vi "niRFUtil FTW Generate RBW FIR Filter.vi"(0 "Type":T2=enum."Gaussian", 5 "Bandwidth (Hz)":T5=500000.0 format="%^.3e", 7 "Sampling Rate (Hz)":dbl=500000.0 format="%^.3e", 9 "Minimum Selectivity (dB)":dbl=70.0 format="%.2f", 11 "Alpha":T1=0.22 format="%.3g") -> (4 "Filter":T3 {"y" min=0 max=127 format="%.2f"; "dx" format="%^.2e"; "x0" format="%^.2e"})   [LabVIEW 2015, in "niRFUtil.lvlib"]
doc: "(c) Copyright 2006, National Instruments, Inc. This VI may not be duplicated, sold, or distributed without written consent from National Instruments."
uses:
  niRFUtil.lvlib
  Includes/niRFUtil INC RBW Filter Bandwidth.ctl
  Includes/niRFUtil INC Real Waveform.ctl
  Includes/niRFUtil INC Real Array.ctl
  Includes/niRFUtil INC RBW Filter Type (Time Domain).ctl
  Includes/niRFUtil INC RRC Filter Alpha.ctl
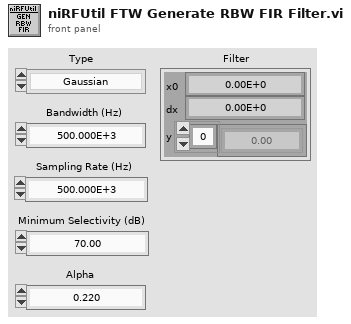
[diagram p1: front panel]
types:
  T1 = typedef "niRFUtil.lvlib/niRFUtil INC RRC Filter Alpha.ctl" = dbl
  T2 = typedef "niRFUtil.lvlib/niRFUtil INC RBW Filter Type (Time Domain).ctl" = enum16{"None", "Gaussian", "Flat", "Synch Tuned - 4", "Synch Tuned - 5", "RRC"}
  T3 = typedef "niRFUtil.lvlib/niRFUtil INC Real Waveform.ctl" = cluster{"x0":dbl, "dx":dbl, "y":T4}
  T4 = typedef "niRFUtil.lvlib/niRFUtil INC Real Array.ctl" = sgl[]
  T5 = typedef "niRFUtil.lvlib/niRFUtil INC RBW Filter Bandwidth.ctl" = dbl
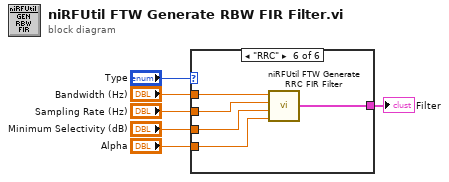
[diagram p0: block diagram]
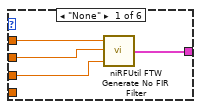
[diagram p2: hidden frame]
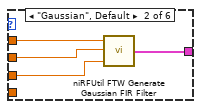
[diagram p3: hidden frame]
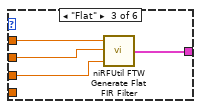
[diagram p4: hidden frame]
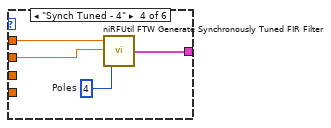
[diagram p5: hidden frame]
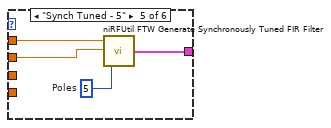
[diagram p6: hidden frame]
diagram:
  n1 = case shown="\"RRC\"" "Type" {
    tunnel: "Bandwidth (Hz)" -> [w10 w14 w18 w22 w26 w31]
    tunnel: "Sampling Rate (Hz)" -> [w9 w13 w17 w21 w25 w30]
    tunnel: "Minimum Selectivity (dB)" -> [w7 w12 w15 _ _ w29]
    tunnel: [w8 w11 w16 w20 w24 w27] -> w2
    tunnel: "Alpha" -> [_ _ _ _ _ w28]
    frame "None" {
      n2 = call "niRFUtil FTW Generate No FIR Filter.vi"("Minimum Selectivity (dB)"=w7, "Sampling Rate (Hz)"=w9, "Bandwidth (Hz)"=w10) -> ("Filter"=w8:T3)
    }
    frame "Gaussian", Default {
      n3 = call "niRFUtil FTW Generate Gaussian FIR Filter.vi"("Minimum Selectivity (dB)"=w12, "Sampling Rate (Hz)"=w13, "Bandwidth (Hz)"=w14) -> ("Filter"=w11:T3)
    }
    frame "Flat" {
      n4 = call "niRFUtil FTW Generate Flat FIR Filter.vi"("Minimum Selectivity (dB)"=w15, "Sampling Rate (Hz)"=w17, "Bandwidth (Hz)"=w18) -> ("Filter"=w16:T3)
    }
    frame "Synch Tuned - 4" {
      w19 = 4  # Poles
      n5 = call "niRFUtil FTW Generate Synchronously Tuned FIR Filter.vi"("Poles (5)"=w19, "Sampling Rate (Hz)"=w21, "RBW (Hz)"=w22) -> ("Filter"=w20:T3)
    }
    frame "Synch Tuned - 5" {
      w23 = 5  # Poles
      n6 = call "niRFUtil FTW Generate Synchronously Tuned FIR Filter.vi"("Poles (5)"=w23, "Sampling Rate (Hz)"=w25, "RBW (Hz)"=w26) -> ("Filter"=w24:T3)
    }
    frame "RRC" {
      n7 = call "niRFUtil FTW Generate RRC FIR Filter.vi"("Alpha"=w28, "Minimum Selectivity (dB)"=w29, "Sampling Rate (Hz)"=w30, "Bandwidth (Hz)"=w31) -> ("Filter"=w27:T3)
    }
  }
  "Filter" <- w2
